vi "WriteIOSafeCondition b2g2.vi"(1 "error in":errorcluster) -> (0 "error out":errorcluster)   [LabVIEW 2011]
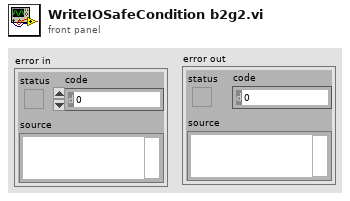
[diagram p1: front panel]
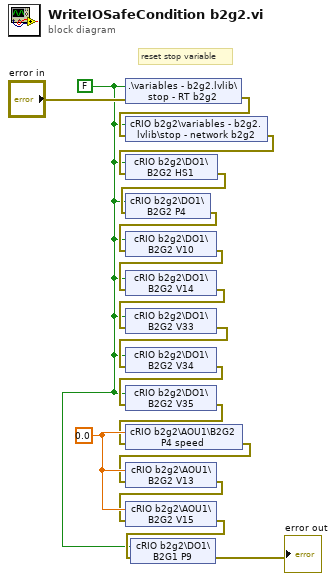
[diagram p0: block diagram]
diagram:
  w1 = FALSE ("B2G1 P-4")
  w16 = 0.0 ("B2G1 V-13")
  # "reset stop variable"
  n1 = shared-variable ".\\variables - b2g2.lvlib\\stop - RT b2g2"(w1, error in="error in") -> (error out=w14:errorcluster)
  n2 = shared-variable "cRIO b2g2\\variables - b2g2.lvlib\\stop - network b2g2"(w1, error in=w14) -> (error out=w13:errorcluster)
  n3 = shared-variable "cRIO b2g2\\DO1\\B2G2 HS1"(w1, error in=w13) -> (error out=w12:errorcluster)
  n4 = shared-variable "cRIO b2g2\\DO1\\B2G2 P4"(w1, error in=w12) -> (error out=w4:errorcluster)
  n5 = shared-variable "cRIO b2g2\\DO1\\B2G2 V10"(w1, error in=w4) -> (error out=w5:errorcluster)
  n6 = shared-variable "cRIO b2g2\\DO1\\B2G2 V14"(w1, error in=w5) -> (error out=w6:errorcluster)
  n7 = shared-variable "cRIO b2g2\\DO1\\B2G2 V33"(w1, error in=w6) -> (error out=w7:errorcluster)
  n8 = shared-variable "cRIO b2g2\\DO1\\B2G2 V34"(w1, error in=w7) -> (error out=w8:errorcluster)
  n9 = shared-variable "cRIO b2g2\\DO1\\B2G2 V35"(w1, error in=w8) -> (error out=w9:errorcluster)
  n10 = shared-variable "cRIO b2g2\\AOU1\\B2G2 P4 speed"(w16, error in=w9) -> (error out=w10:errorcluster)
  n11 = shared-variable "cRIO b2g2\\AOU1\\B2G2 V13"(w16, error in=w10) -> (error out=w11:errorcluster)
  n12 = shared-variable "cRIO b2g2\\AOU1\\B2G2 V15"(w16, error in=w11) -> (error out=w2:errorcluster)
  n13 = shared-variable "cRIO b2g2\\DO1\\B2G1 P9"(w1, error in=w2) -> (error out=→"error out":errorcluster)
